vi "test 9401 DIO Scan Mode Loop Back.vi"(8 "error in (no error)":errorcluster, 11 "TestCase in":refnum<class "Scan Engine EtherCAT System Tests.lvclass">) -> (0 "error out":errorcluster, 3 "TestCase out":refnum<class "Scan Engine EtherCAT System Tests.lvclass">)   [LabVIEW 2017, in "Scan Engine EtherCAT System Tests.lvclass"]
uses:
  Scan Engine EtherCAT System Tests.lvclass
  C:/Users/nitest/Desktop/Git/niveristand-custom-device-testing-tools/VeriStandTestCase/VeriStandTestCase.lvclass
  <vilib>/addons/_JKI Toolkits/VI Tester/TestCase.llb/TestCase.lvclass
  niveristand-custom-device-testing-tools/VeriStandTestCase/VeriStandTestCase.lvclass
  C:/Program Files (x86)/National Instruments/LabVIEW 2017/vi.lib/addons/_JKI Toolkits/VI Tester/TestCase.llb/TestCase.lvclass
  Scan Engine Custom Device.lvlib
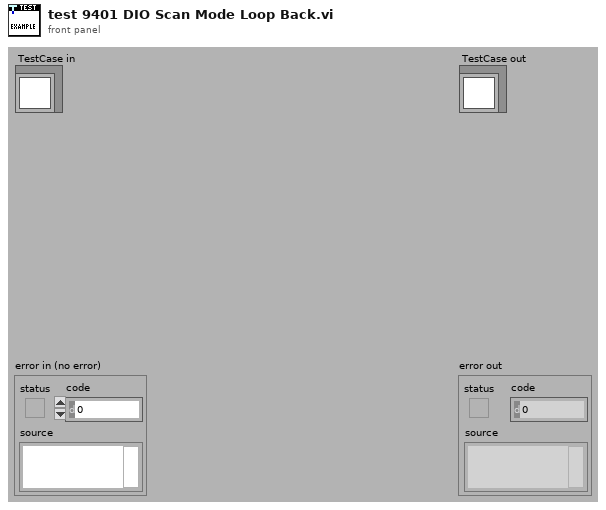
[diagram p1: front panel]
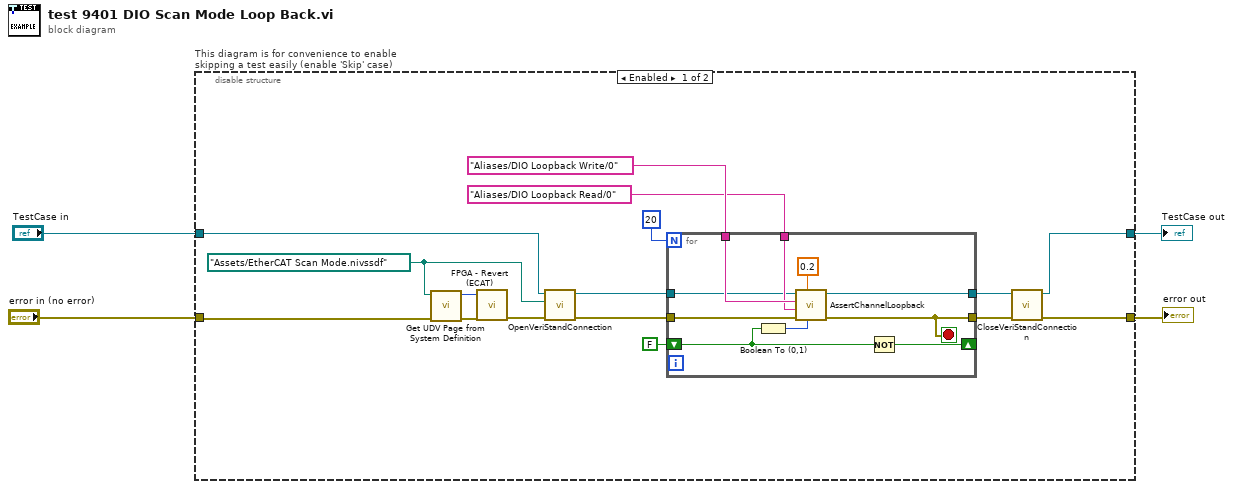
[diagram p0: block diagram]
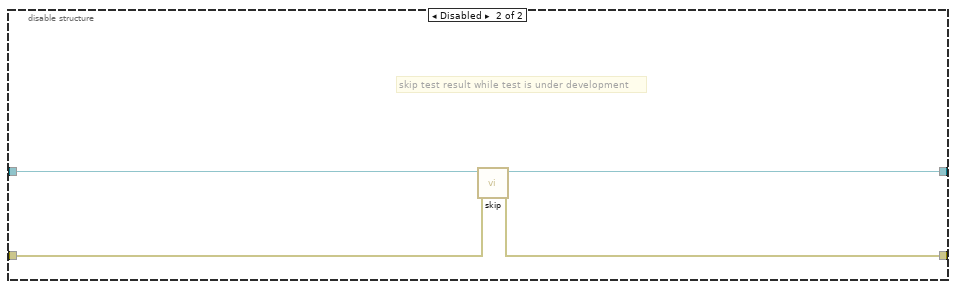
[diagram p2: hidden frame]
diagram:
  n1 = disable-structure "This diagram is for convenience to enable skipping a test easily (enable 'Skip' case)" shown="Enabled" {
    disable-tunnel: "TestCase in" -> [w14 w34]
    disable-tunnel: [w10 w32] -> w1
    disable-tunnel: [w11 w33] -> w3
    disable-tunnel: "error in (no error)" -> [w7 w31]
    frame Enabled {
      w6 = path "Assets/EtherCAT Scan Mode.nivssdf" ("System Definition File")
      n2 = call "Get UDV Page from System Definition.vi"("error in (no error)"=w7, "System Definition Path"=w6) -> ("error out"=w8:errorcluster, "NodeID"=w5:u64)  [unwired: 8 in]
      n3 = call "FPGA - Revert (ECAT).vi"("error in (no error)"=w8, "Node Ptr"=w5) -> ("error out"=w9:errorcluster)  [unwired: 9 in]
      n4 = call-dynamic "OpenVeriStandConnection.vi"("error in (no error)"=w9, "System Definition File"=w6, "VeriStand Test Case in"=w14) -> ("error out"=w16:errorcluster, "VeriStand Test Case out"=w15:refnum<class "Scan Engine EtherCAT System Tests.lvclass">)  [unwired: 6 in, 1 out]
      n5 = for {
        N: 20 -> [_]
        tunnel: "Aliases/DIO Loopback Write/0" ("Channel") -> [w27]
        tunnel: [w25] -> w13
        tunnel: "Aliases/DIO Loopback Read/0" ("Channel") -> [w26]
        shift-right: [w30] -> _
        shift-left: FALSE -> [w29]
        tunnel: w16 -> [w28]
        tunnel: [w22] -> w12
        tunnel: w15 -> [w23]
        stop <- w25 stop-if-true
        n6 = Boolean To (0,1)(Boolean=w29) -> (0, 1=w24:i16)
        n7 = call "AssertChannelLoopback.vi"("Value"=w24, "Delay Time (s)"=0.2, "error in (no error)"=w28, "Read Channel"=w26, "Write Channel"=w27, "VeriStand Test Case in"=w23) -> ("error out"=w25:errorcluster, "VeriStand Test Case out"=w22:refnum<class "Scan Engine EtherCAT System Tests.lvclass">)  [unwired: 4 in]
        n8 = Not(x=w29) -> (.not. x?=w30:bool)
      }
      n9 = call-dynamic "CloseVeriStandConnection.vi"("error in (no error)"=w13, "VeriStand Test Case in"=w12) -> ("error out"=w11:errorcluster, "VeriStand Test Case out"=w10:refnum<class "Scan Engine EtherCAT System Tests.lvclass">)  [unwired: 8 in]
    }
    frame Disabled {
      # "skip test result while test is under development"
      n10 = call <vilib>:"skip.vi"("error in (no error)"=w31, "TestCase in"=w34) -> ("error out"=w33:errorcluster, "TestCase out"=w32:refnum<class "Scan Engine EtherCAT System Tests.lvclass">)  [unwired: 8 in]
    }
  }
  "error out" <- w3
  "TestCase out" <- w1
